vi "Chamber controller Dec 2 2016 new turbo - biased QCM.vi"() -> ()   [LabVIEW 2014]
uses:
  <vilib>/Instr/_visa.llb/VISA Configure Serial Port (Instr).vi
  Environmental Chamber LabVIEW and Instruments/Drivers and Software/Keithley 2100 Series/Public/Configure/Configure 2 Wire Resistance.vi
  <vilib>/Utility/file.llb/Write To Spreadsheet File (string).vi
  <vilib>/Utility/file.llb/Read From Spreadsheet File (string).vi
  Environmental Chamber LabVIEW and Instruments/Drivers and Software/keithley_6430/Keithley 6430/Public/Data/Read (Single Point).vi
  Environmental Chamber LabVIEW and Instruments/Drivers and Software/LabVIEW 8.2 Drivers/keithley_24xx/Keithley 24XX/Public/Data/Read (Single Point).vi
  Environmental Chamber LabVIEW and Instruments/Drivers and Software/keithley_24xx/Keithley 24XX/Keithley 24XX.lvlib
  Environmental Chamber LabVIEW and Instruments/Drivers and Software/keithley_6430/Keithley 6430/Keithley 6430.lvlib
  Environmental Chamber LabVIEW and Instruments/Drivers and Software/Keithley 2100 Series/Keithley 2100 Series.lvlib
panel:
  out "SRS freq plot":dbl(graph)
  out "Numeric bias":dbl
  out "bias voltage":string
  out "Current":sgl
  out "Resistance":sgl
  in  "Applied Voltage (V)":dbl min=-5.0 max=5.0 step=5e-06
  in  "Arduino COMs":T1={"Arduino 1"="COM23", "Arduino 2"="COM24", "Arduino 3"="COM25", "Arduino 4"="COM26", "Arduino 5"="COM27", "Arduino 6"="COM28"}
  out "saving data?":bool
  out "ArduinoQCM\ncluster":T2 caption="Arduino QCM" {"6" format="%_8g"; "5" format="%_8g"; "4" format="%_8g"; "3" format="%_8g"; "2" format="%_8g"; "1" format="%#_10g"}
  in  "Data logging settings":T3={"Save during sequence only"=TRUE, "Save now"=FALSE, "sec between data points"=0.0, "Current data file path"=path "", "Save sample names"={"QCM1"="", "QCM2"="", "QCM3"="", "QCM4"="", "QCM5"="", "QCM6"="", "SRS"="", "K-2420"="", "K-6430"="", "K-2100"=""}, "Experiment Notes"=""} {"sec between data points" min=0.0 max=30.0 format="%#_13g"}
  in  "Sequence cluster":T4={"Save sequence"=FALSE, "Clear sequence"=FALSE, "Import sequence file"=FALSE, "Tare elapsed time"=TRUE, "Run Sequence"=FALSE, "Stop program when sequence ends"=TRUE, "User-defined\nsequence"=[], "Sequence end time"="", "Sequence\npreview"=[], "Current\nstep"=0} caption="Sequence settings"
  in  "Pressure parameters cluster":T5={"valve % open"=100.0, "Desired pressure"=0.0, "Vapor sccm"=0.0, "Gas sccm"=0.0, "Valve mode"=enum."% Open", "Pressure Mode"=enum."Abs. pressure", "analyte partial pressure"=23.8, "Turbo pump\nauto on"=TRUE, "Valve position (%)"=0.0, "read pressure"=0.0, "read vapor flow"=0.0, "read gas flow"=0.0, "pressure chart"={"pressure"=0.0}} caption="Pressure settings" {"read gas flow" format="%#_3g"; "read vapor flow" format="%#_3g"; "read pressure" format="%#_7f"; "Valve position (%)" format="%#_3g"; "analyte partial pressure" min=0.0 max=100.0 step=5.0; "Gas sccm" min=0 max=200 step=5; "Vapor sccm" min=0 max=200 step=5; "Desired pressure" min=0.0 max=760.0 step=5.0; "valve % open" min=0.0 max=100.0 step=5.0 format="%#_2f"}
  out "J-KEM temp chart":dbl(graph)
  out "Elapsed time (min)":dbl
  out "State date/time":string caption="Start time"
  out "K-2100 (Ohm)":cluster{"Measurement":dbl}(graph) caption="K-2100"
  out "K-6430":cluster{"Measurement":dbl}(graph)
  out "K-2420":cluster{"Applied Voltage (V)":dbl}(graph)
  in  "Gate time (sec)":enum16{"0.1", "1.0 ", "10"}(ring)=enum."1.0 "
  out "Hz":dbl format="%#.7f"
  out "QCM plot":T6(graph)
  in  "Stop":bool
  in  "Clear all charts":bool
  out "O2 sensor output":dbl[](array[numeric]) caption="atm\nTorr"
  in  "rapidox O2 Sensor":bool
  in  "setnag O2 Pump":bool
  in  "Baud Rate 2":i32(ring)=2 items=["2400", "4800", "9600", "19200", "38400", "57600", "115200"]
  in  "Com Port":i32(ring) items=["Com 1", "Com 2", "Com 3", "Com 4", "Com 5", "Com 6", "COM 7", "COM 8", "COM 9", "COM 10", "COM 11", "COM 12", "com 13", "COM 14"]
  in  "Com Port 2":i32(ring) items=["Com 1", "Com 2", "Com 3", "Com 4", "Com 5", "Com 6", "COM 7", "COM 8", "COM 9", "COM 10", "COM 11", "COM 12", "com 13", "COM 14"]
  out "Waveform Chart":cluster{dbl}(graph)
  out "O2 Concentration (PPM)":dbl
  out "Waveform Chart 6":cluster{dbl}(graph)
  # "SRS"
  # "Currently Unused"
  # "100%"
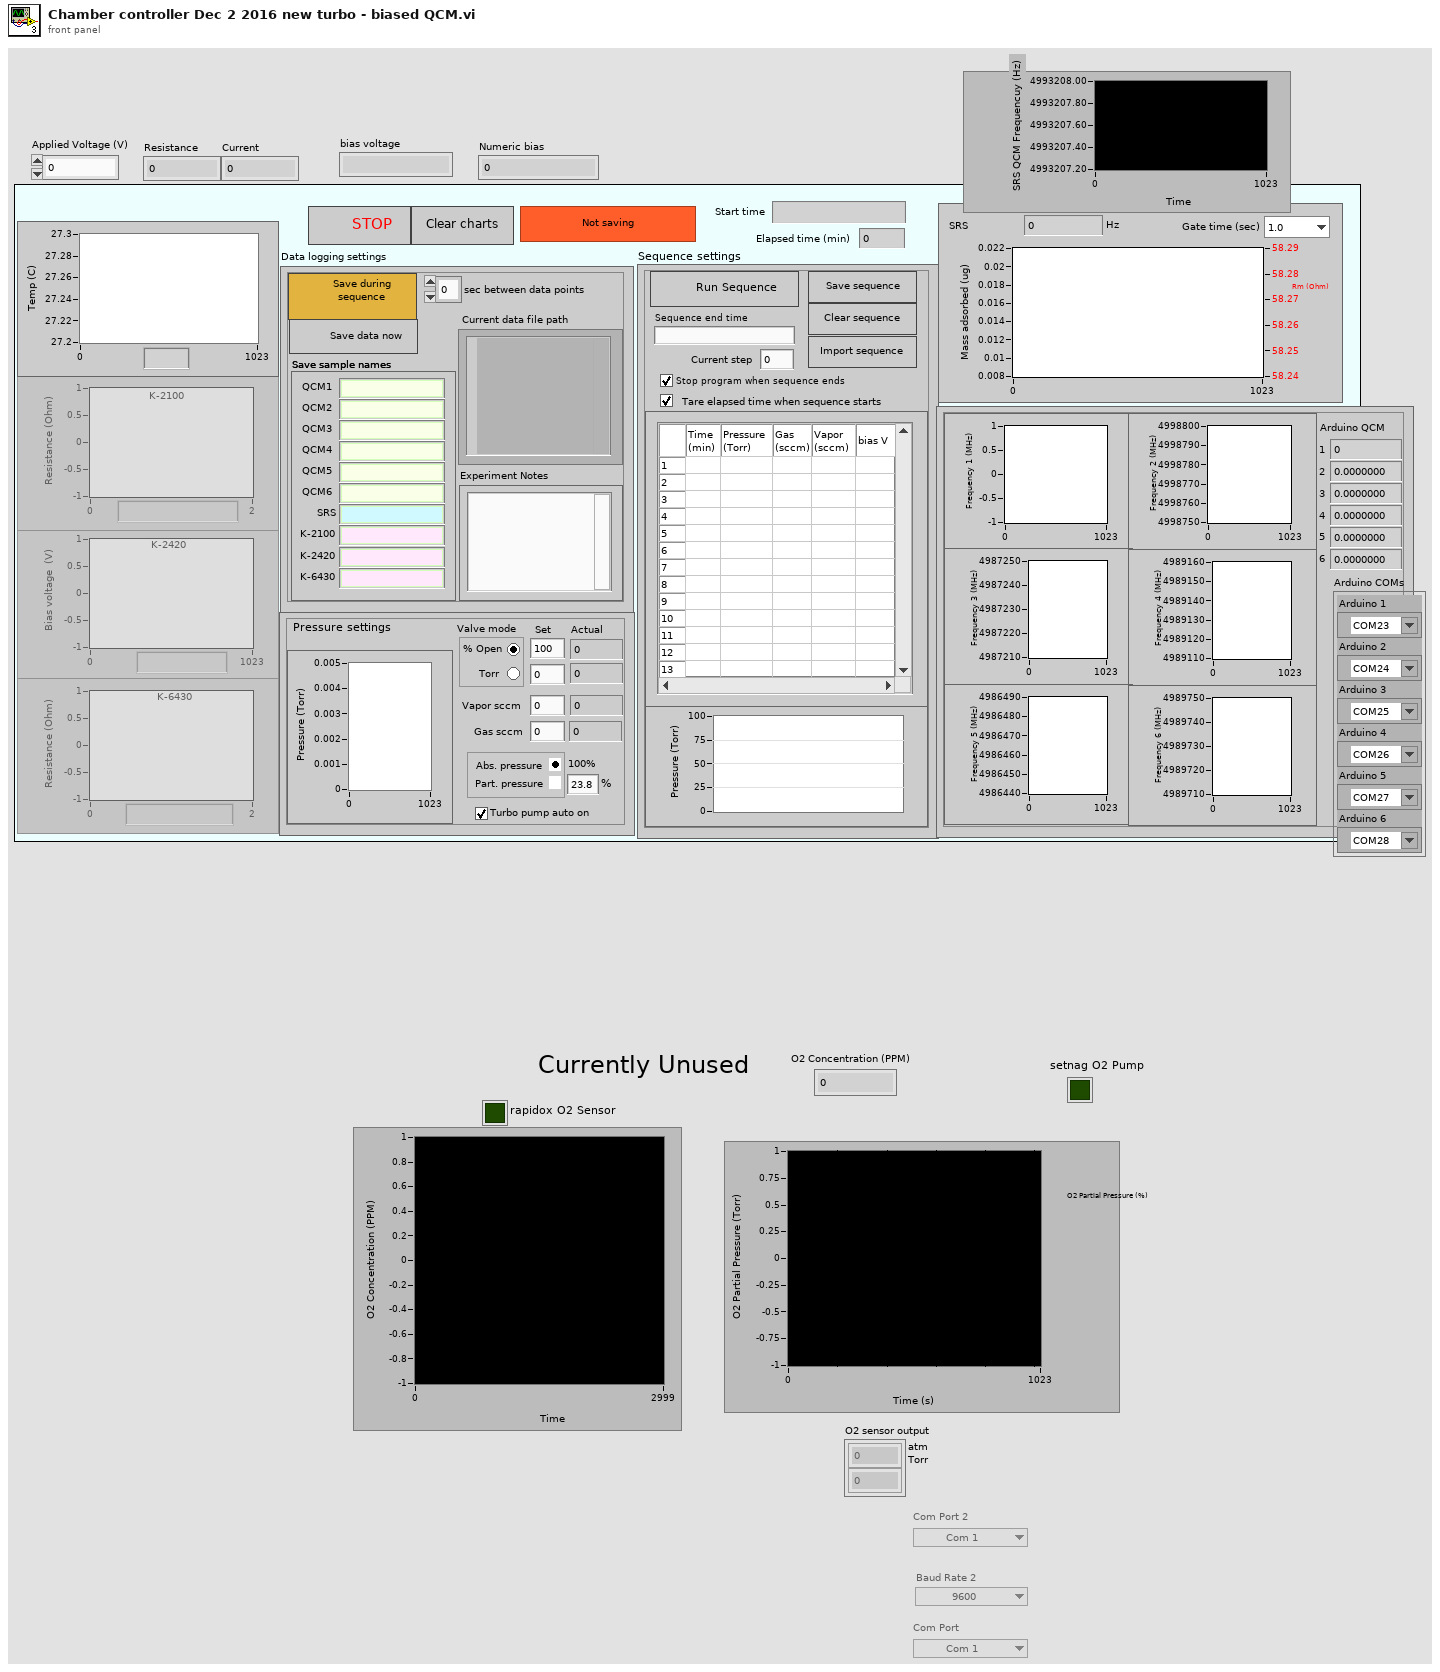
[diagram p1: front panel]
types:
  T1 = cluster{"Arduino 1":refnum<visa-resource-name>, "Arduino 2":refnum<visa-resource-name>, "Arduino 3":refnum<visa-resource-name>, "Arduino 4":refnum<visa-resource-name>, "Arduino 5":refnum<visa-resource-name>, "Arduino 6":refnum<visa-resource-name>}
  T2 = cluster{"arduino qcm 1":dbl, "1":dbl, "arduino qcm 2":dbl, "2":dbl, "arduino qcm 3":dbl, "3":dbl, "arduino qcm 4":dbl, "4":dbl, "arduino qcm 5":dbl, "5":dbl, "arduino qcm 6":dbl, "6":dbl}
  T3 = cluster{"Save during sequence only":bool, "Save now":bool, "sec between data points":dbl, "Current data file path":path, "Save sample names":cluster{"QCM1":string, "QCM2":string, "QCM3":string, "QCM4":string, "QCM5":string, "QCM6":string, "SRS":string, "K-2420":string, "K-6430":string, "K-2100":string}, "Experiment Notes":string}
  T4 = cluster{"Save sequence":bool, "Clear sequence":bool, "Import sequence file":bool, "Tare elapsed time":bool, "Run Sequence":bool, "Stop program when sequence ends":bool, "User-defined\nsequence":string[][], "Sequence end time":string, "Sequence\npreview":cluster{dbl[], dbl[]}[], "Current\nstep":i32}
  T5 = cluster{"valve % open":dbl, "Desired pressure":dbl, "Vapor sccm":sgl, "Gas sccm":sgl, "Valve mode":enum32{"% Open", "Torr "}, "Pressure Mode":enum32{"Abs. pressure", " Part. pressure"}, "analyte partial pressure":dbl, "Turbo pump\nauto on":bool, "Valve position (%)":dbl, "read pressure":dbl, "read vapor flow":dbl, "read gas flow":dbl, "pressure chart":cluster{"pressure":dbl}}
  T6 = cluster{"Numeric Control":dbl, "Resistance out":dbl}
  T7 = cluster{"Keithley 6430":bool, "J-KEM":bool, "Keithley 2420":bool, "Keithley 2100":bool, "SRS QCM":bool, "Pressure control":bool, "Arduino":bool}
  T8 = enum8{"Enabled", "Disabled", "Disabled and Grayed Out"}
  T9 = enum16{"open", "open or create", "create or replace", "create", "open (read only)"}
  T10 = enum16{"no parity", "odd parity", "even parity", "mark parity", "space parity"}
  T11 = cluster{"String":string, "String":string, "String":string}
  T12 = cluster{bool, "task out":refnum<k21>, "error out":errorcluster, "task out":refnum<k21>, "error out":errorcluster, "turbo pump":refnum<visa-resource-name>, "error out":errorcluster}
  T13 = cluster{bool, "task out":refnum<k21>, "error out":errorcluster, "task out":refnum<k21>, "error out":errorcluster, "VISA resource name out":refnum<visa-resource-name>, "error out":errorcluster}
  T14 = cluster{bool, "VISA resource name":refnum<visa-resource-name>, "error out":errorcluster}
  T15 = cluster{bool, "VISA resource name out":refnum<visa-resource-name>, "error out":errorcluster}
  T16 = cluster{"VISA resource name out":refnum<visa-resource-name>, "error out":errorcluster, "VISA resource name out":refnum<visa-resource-name>, "error out":errorcluster, "VISA resource name out":refnum<visa-resource-name>, "error out":errorcluster, "VISA resource name out":refnum<visa-resource-name>, "error out":errorcluster, "VISA resource name out":refnum<visa-resource-name>, "error out":errorcluster, "VISA resource name out 2":refnum<visa-resource-name>, "error out 2":errorcluster}
  T17 = cluster{"Boolean":bool, "VISA resource name out":refnum<visa-resource-name>, "error out":errorcluster}
  T18 = cluster{bool, "VISA out":refnum<visa-resource-name>, "error out":errorcluster}
  T19 = cluster{"Boolean":bool, "VISA out":refnum<visa-resource-name>, "error out":errorcluster}
  T20 = cluster{"Numeric Control":dbl, "Cluster":cluster{"Numeric Control":dbl}, "String":string, "error out":errorcluster}
  T21 = cluster{bool, "Com Port":i32, "Numeric Control out":dbl}
  T22 = cluster{"Arduino address":refnum<visa-resource-name>, "error in (no error)":errorcluster, "Arduino address 2":refnum<visa-resource-name>, "error in (no error) 2":errorcluster, "Arduino address 3":refnum<visa-resource-name>, "error in (no error) 3":errorcluster, "Arduino address 4":refnum<visa-resource-name>, "error in (no error) 4":errorcluster, "Arduino address 5":refnum<visa-resource-name>, "error in (no error) 5":errorcluster, "Arduino address 6":refnum<visa-resource-name>, "error in (no error) 6":errorcluster}
  T23 = cluster{"mean":string, "mean":string, "mean":string, "mean":string, "mean":string, "mean":string}
  T24 = cluster{"valve % open":dbl, "Desired pressure":dbl, "Vapor sccm":sgl, "Gas sccm":sgl, "Valve mode":enum32{"% Open", "Torr "}, "Pressure Mode":enum32{"Abs. pressure", " Part. pressure"}, "analyte partial pressure":dbl}
  T25 = cluster{"User-defined\nsequence":string[][], "Present (s)":dbl, "current  step # in":i32, "sequence end time in":timestamp}
  T26 = cluster{"current  step # in":i32, "sequence end time in":timestamp, "Boolean":bool}
  T27 = cluster{"press/RH/gas/vapor":cluster{"pressure":string, "RH":string, "gas flow":string, "vapor flow":string}, "Cluster":cluster{"Valve position (%)":dbl, "read pressure":dbl, "read vapor flow":dbl, "read gas flow":dbl}}
  T28 = cluster{"Boolean":bool, "task out":refnum<k21>, "error out":errorcluster, "task out":refnum<k21>, "error out":errorcluster, "VISA resource name out":refnum<visa-resource-name>, "error out":errorcluster}
  T29 = cluster{"f":dbl, "f":dbl, "f":dbl, "f":dbl, "f":dbl}[]
  T30 = cluster{"pressure":string, "RH":string, "gas flow":string, "vapor flow":string}
  T31 = cluster{"Valve position (%)":dbl, "read pressure":dbl, "read vapor flow":dbl, "read gas flow":dbl}
  T32 = cluster{"mean":dbl, "mean":dbl, "mean":dbl, "mean":dbl, "mean":dbl, "mean":dbl}
  T33 = cluster{"QCM1":string, "QCM2":string, "QCM3":string, "QCM4":string, "QCM5":string, "QCM6":string, "SRS":string, "K-2420":string, "K-6430":string, "K-2100":string}
  T34 = cluster{"mean":dbl, "mean":dbl, "mean":dbl, "mean":dbl, "mean":dbl, "mean":dbl, "mean":dbl, "mean":dbl, "mean":dbl, "mean":dbl, "mean":dbl, "mean":dbl}
  T35 = cluster{"String data out":string, string, string, string}
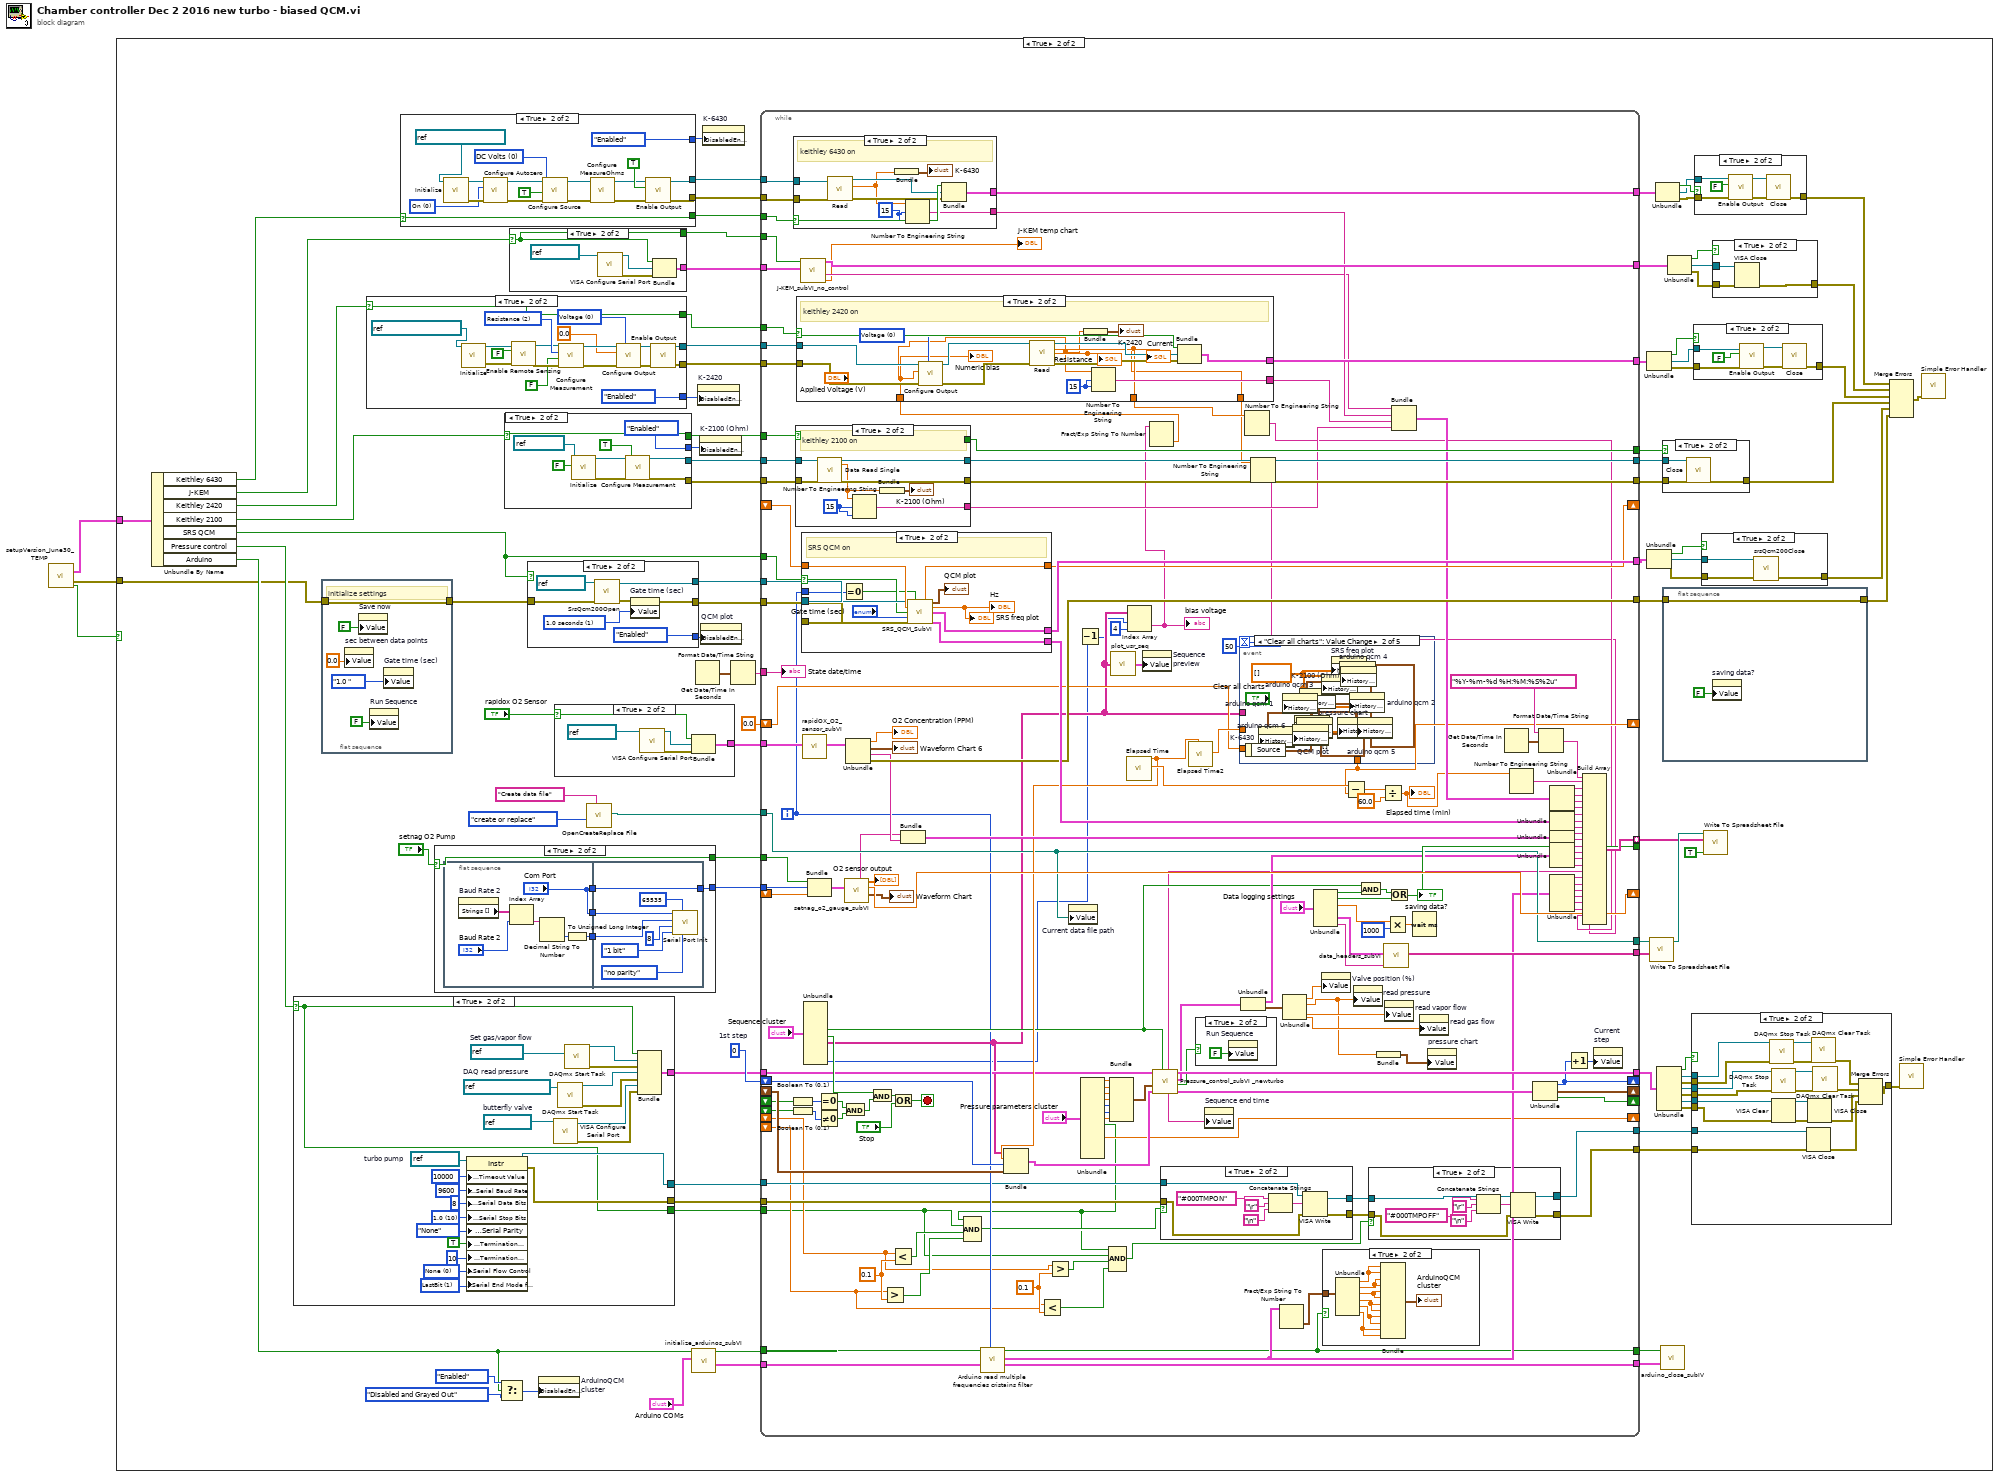
[diagram p0: block diagram]
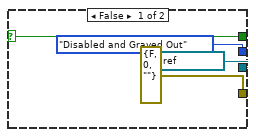
[diagram p4: hidden frame]
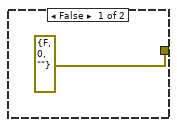
[diagram p5: hidden frame]
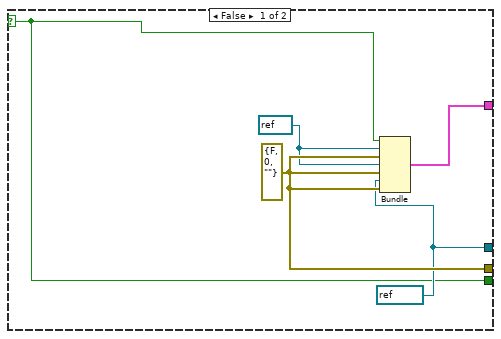
[diagram p6: hidden frame]
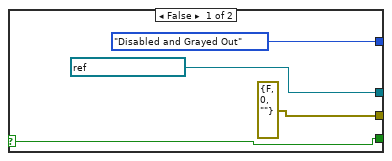
[diagram p8: hidden frame]
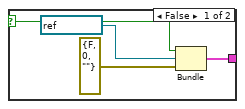
[diagram p9: hidden frame]
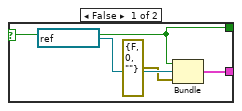
[diagram p11: hidden frame]
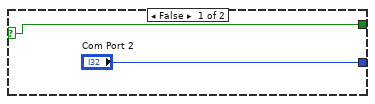
[diagram p12: hidden frame]
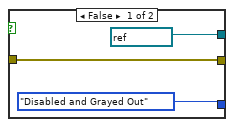
[diagram p14: hidden frame]
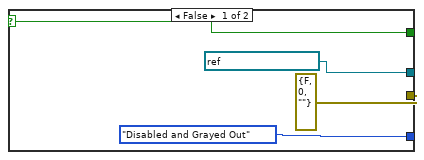
[diagram p16: hidden frame]
diagram:
  n1 = call "setupVersion_June30_TEMP.vi"() -> ("Instruments on/off"=w1:T7, "error IO"=w2:errorcluster, "OK"=w3:bool)  [unwired: 13 in]
  n2 = case shown="True" w3 {
    tunnel: w2 -> [_ w17]
    tunnel: w1 -> [_ w27]
    frame False {
    }
    frame True {
      w34 = 0  # 1st step
      n3 = Unbundle By Name(w27) -> ("Keithley 6430"=w26:bool, "J-KEM"=w25:bool, "Keithley 2420"=w24:bool, "Keithley 2100"=w23:bool, "SRS QCM"=w22:bool, "Pressure control"=w21:bool, "Arduino"=w20:bool)
      n4 = case shown="True" w21 {
        selector: w21 -> [w142 w147]
        tunnel: [w146 w148] -> w15
        tunnel: [w145 w150] -> w7
        tunnel: [w143 w149] -> w8
        tunnel: [w142 w147] -> w6
        frame False {
          w143 = refnum<visa-resource-name> refnum ("turbo pump")
          w144 = refnum<k21> refnum ("task out")
          w145 = errorcluster {"status"=FALSE, "code"=0, "source"=""} ("error out")
          n5 = Bundle(w142, "task out"=w144, "error out"=w145, "task out"=w144, "error out"=w145, "turbo pump"=w143, "error out"=w145) -> (w146:T12)  [unwired: 1 in]
        }
        frame True {
          w154 = u16 1 items=["None", "LastBit", "TermChar"] ("Serial Settings:Serial End Mode for Reads")
          w152 = u16 0 items=["None", "XON/XOFF", "RTS/CTS", "XON/XOFF & RTS/CTS", "DTR/DSR", "XON/XOFF & DTR/DSR"] ("flow control (0:none)")
          w155 = u16 10 items=["1.0"=10, "1.5"=15, "2.0"=20] ("stop bits (10: 1 bit)")
          w151 = refnum<visa-resource-name> "COM7"  # turbo pump
          w167 = refnum<visa-resource-name> "COM5"  # butterfly valve
          w168 = refnum<k21> "Setflow"  # Set gas/vapor flow
          w169 = refnum<k21> "AllDaqReadings"  # DAQ read pressure
          n6 = property class="Instr"(reference=w151, "General Settings:Timeout Value"=u32 10000 ("timeout (10sec)"), "Serial Settings:Serial Baud Rate"=u32 9600 ("baud rate (9600)"), "Serial Settings:Serial Data Bits"=u16 8 ("data bits (8)"), "Serial Settings:Serial Stop Bits"=w155, "Serial Settings:Serial Parity"=enum16{"None", "Odd", "Even", "Mark", "Space"}."None" ("parity (0:none)"), "Message Based Settings:Termination Character Enable"=TRUE ("Enable Termination\nChar (T)"), "Message Based Settings:Termination Character"=u8 10 ("termination char\n(0xA = '\\n' = LF)"), "Serial Settings:Serial Flow Control"=w152, "Serial Settings:Serial End Mode for Reads"=w154) -> (reference out=w149:refnum<visa-resource-name>, error out=w150:errorcluster)  [unwired: 1 in]
          n7 = call-poly "VISA Configure Serial Port"("VISA resource name"=w167) -> ("VISA resource name out"=w162:refnum<visa-resource-name>, "error out"=w161:errorcluster)  [unwired: 13 in]
          n8 = call <vilib>:"DAQmx Start Task.vi"("task/channels in"=w169) -> ("task out"=w164:refnum<k21>, "error out"=w163:errorcluster)  [unwired: 13 in]
          n9 = call <vilib>:"DAQmx Start Task.vi"("task/channels in"=w168) -> ("task out"=w166:refnum<k21>, "error out"=w165:errorcluster)  [unwired: 13 in]
          n10 = Bundle(w147, "task out"=w166, "error out"=w165, "task out"=w164, "error out"=w163, "VISA resource name out"=w162, "error out"=w161) -> (w148:T13)  [unwired: 1 in]
        }
      }
      n11 = flat-sequence {
        tunnel: [w98] -> w16
        tunnel: w17 -> [w98]
        frame #0 {
          # "initialize settings"
          n12 = property on="sec between data points" class="DigNum (strict)"("Value"=0.0) -> ()  [unwired: 2 in, 2 out]
          n13 = property on="Save now" class="Bool (strict)"("Value"=FALSE) -> ()  [unwired: 2 in, 2 out]
          n14 = property on="Run Sequence" class="Bool (strict)"("Value"=FALSE) -> ()  [unwired: 2 in, 2 out]
          n15 = property on="Gate time (sec)" class="Enum (strict)"("Value"=enum16{"0.1", "1.0 ", "10"}."1.0 " ("Gate time (sec)")) -> ()  [unwired: 2 in, 2 out]
        }
      }
      n16 = case shown="True" w24 {
        selector: w24 -> [w261 w265]
        tunnel: [refnum<visa-resource-name> "GPIB1::24::INSTR" ("VISA resource name") w274] -> w95
        tunnel: [errorcluster {"status"=FALSE, "code"=0, "source"=""} ("error out") w269] -> w94
        tunnel: [T8."Disabled and Grayed Out" ("Disabled") T8."Enabled" ("Disabled")] -> w58
        tunnel: [w261 w265] -> w51
        frame False {
        }
        frame True {
          w276 = u16 0 items=["Voltage", "Current"] ("Source Mode  (0: Voltage)")
          w281 = u16 2 items=["Volts", "Current", "Resistance"] ("Function (0: Volts)")
          n17 = call "Initialize.vi"("VISA resource name"=refnum<visa-resource-name> "GPIB1::24::INSTR") -> ("error out"=w270:errorcluster, "VISA resource name out"=w273:refnum<visa-resource-name>)  [unwired: 9 in]
          n18 = call "Enable Remote Sensing.vi"("error in (no error)"=w270, "Enable Remote Sensing (T: Enable)"=FALSE ("4-wire?"), "VISA resource name"=w273) -> ("error out"=w271:errorcluster, "VISA resource name out"=w272:refnum<visa-resource-name>)  [unwired: 7 in]
          n19 = call "Configure Measurement.vi"("error in (no error)"=w271, "Enable Auto Range (T:Enable)"=FALSE, "Function (0: Volts)"=w281, "VISA resource name"=w272) -> ("error out"=w280:errorcluster, "VISA resource name out"=w279:refnum<visa-resource-name>)  [unwired: 6 in]
          n20 = call "Configure Output.vi"("Source Mode  (0: Voltage)"=w276, "error in (no error)"=w280, "Output Level (0)"=0.0 ("Applied Voltage (V)"), "VISA resource name"=w279) -> ("error out"=w278:errorcluster, "VISA resource name out"=w277:refnum<visa-resource-name>)  [unwired: 6 in]
          n21 = call "Enable Output.vi"("error in (no error)"=w278, "VISA resource name"=w277) -> ("error out"=w269:errorcluster, "VISA resource name out"=w274:refnum<visa-resource-name>)  [unwired: 8 in]
        }
      }
      n22 = case shown="True" w26 {
        selector: w26 -> [w177 w181]
        tunnel: [refnum<visa-resource-name> "GPIB0::29::INSTR" ("VISA resource name") w192] -> w64
        tunnel: [errorcluster {"status"=FALSE, "code"=0, "source"=""} ("error out") w193] -> w63
        tunnel: [T8."Disabled and Grayed Out" ("Disabled") T8."Enabled" ("Disabled")] -> w57
        tunnel: [w177 w181] -> w50
        frame False {
        }
        frame True {
          w182 = u16 0 items=["DC Volts", "DC Current"] ("Source Function (0: DC Volts)")
          w189 = u16 0 items=["On", "Off", "Once"] ("Autozero  (0: On)")
          n23 = call "Initialize.vi"("VISA resource name"=refnum<visa-resource-name> "GPIB0::29::INSTR") -> ("error out"=w190:errorcluster, "VISA resource name out"=w191:refnum<visa-resource-name>)  [unwired: 4 in, 5 out]
          n24 = call "Configure Autozero.vi"("error in (no error)"=w190, "Autozero  (0: On)"=w189, "VISA resource name"=w191) -> ("error out"=w185:errorcluster, "VISA resource name out"=w187:refnum<visa-resource-name>)  [unwired: 7 in]
          n25 = call "Configure Source.vi"("error in (no error)"=w185, "Auto Range (T:Enable)"=TRUE, "Source Function (0: DC Volts)"=w182, "VISA resource name"=w187) -> ("error out"=w184:errorcluster, "VISA resource name out"=w186:refnum<visa-resource-name>)  [unwired: 6 in]
          n26 = call "Configure MeasureOhms.vi"("error in (no error)"=w184, "VISA resource name"=w186) -> ("error out"=w197:errorcluster, "VISA resource name out"=w195:refnum<visa-resource-name>)  [unwired: 4 in, 4 out]
          n27 = call "Enable Output.vi"("error in (no error)"=w197, "Enable Output (F:Off)"=TRUE ("Output (F:Off)"), "VISA resource name"=w195) -> ("error out"=w193:errorcluster, "VISA resource name out"=w192:refnum<visa-resource-name>)  [unwired: 7 out]
        }
      }
      n28 = case shown="True" "setnag O2 Pump" {
        selector: "setnag O2 Pump" -> [w220 w222]
        tunnel: ["Com Port 2" w223] -> w91
        tunnel: [w220 w222] -> w39
        frame False {
        }
        frame True {
          n29 = flat-sequence {
            tunnel: ["Com Port"] -> w226
            tunnel: [w228] -> w225
            tunnel: ["Com Port"] -> w224
            tunnel: w226 -> [w234]
            tunnel: w225 -> [w233]
            tunnel: w224 -> [w235]
            tunnel: [w235] -> w223
            frame #0 {
              n30 = property on="Baud Rate 2" class="Ring (strict)"() -> ("Strings []"=w230:string[])  [unwired: 2 in, 2 out]
              n31 = Index Array(array=w230, index="Baud Rate 2") -> (element=w231:string)
              n32 = Decimal String To Number(string=w231) -> (number=w229:i32)  [unwired: 2 in, 1 out]
              n33 = To Unsigned Long Integer(number=w229) -> (unsigned 32bit integer=w228:u32)
            }
            frame #1 {
              n34 = call <vilib>:"Serial Port Init.vi"("parity"=T10."no parity", "buffer size"=u16 65535, "stop bits"=enum16{"1 bit", "1.5 bits", "2 bits"}."1 bit", "data bits"=u16 8, "baud rate"=w233, "port number"=w234) -> ()  [unwired: 1 in, 1 out]
            }
          }
        }
      }
      n35 = Select(t=T8."Enabled" ("Disabled"), s=w20, f=T8."Disabled and Grayed Out" ("Disabled")) -> (s? t:f=w31:T8)
      n36 = case shown="True" w23 {
        selector: w23 -> [w110 w115]
        tunnel: [refnum<visa-resource-name> "K-2100" ("VISA resource name out") w118] -> w48
        tunnel: [errorcluster {"status"=FALSE, "code"=0, "source"=""} ("error out") w117] -> w47
        tunnel: [w110 w115] -> w46
        tunnel: [T8."Disabled and Grayed Out" ("Disabled") T8."Enabled" ("Disabled")] -> w41
        frame False {
        }
        frame True {
          n37 = call "Initialize.vi"("VISA resource name"=refnum<visa-resource-name> "K-2100", "Reset? (T: Reset)"=FALSE) -> ("VISA resource name out"=w119:refnum<visa-resource-name>, "error out"=w116:errorcluster)  [unwired: 16 in]
          n38 = call-poly "Configure Measurement.vi"("VISA resource name"=w119, "error in (no error)"=w116, "Auto Range? (T: Auto)"=TRUE) -> ("VISA resource name out"=w118:refnum<visa-resource-name>, "error out"=w117:errorcluster)  [unwired: 15 in]
        }
      }
      n39 = case shown="True" w25 {
        selector: w25 -> [w211 w216]
        tunnel: [w212 w217] -> w80
        tunnel: [w211 w216] -> w74
        frame False {
          n40 = Bundle(w211, "VISA resource name"=refnum<visa-resource-name> "COM3", "error out"=errorcluster {"status"=FALSE, "code"=0, "source"=""}) -> (w212:T14)  [unwired: 1 in]
        }
        frame True {
          n41 = call-poly "VISA Configure Serial Port"("VISA resource name"=refnum<visa-resource-name> "COM3") -> ("VISA resource name out"=w218:refnum<visa-resource-name>, "error out"=w215:errorcluster)  [unwired: 13 in]
          n42 = Bundle(w216, "VISA resource name out"=w218, "error out"=w215) -> (w217:T15)  [unwired: 1 in]
        }
      }
      n43 = case shown="True" w22 {
        tunnel: [refnum<visa-resource-name> "COM6" ("VISA in") w250] -> w93
        tunnel: [w245 w247] -> w92
        tunnel: w16 -> [w245 w252]
        tunnel: [T8."Disabled and Grayed Out" ("Disabled") T8."Enabled" ("Disabled")] -> w59
        frame False {
        }
        frame True {
          w249 = u16 1 items=["0.1 seconds", "1.0 seconds", "10.0 seconds"] ("Gate time")
          n44 = call "SrsQcm200Open.vi"("error in"=w252, "VISA in"=refnum<visa-resource-name> "COM6") -> ("error out"=w248:errorcluster, "VISA out"=w250:refnum<visa-resource-name>)  [unwired: 3 in]
          n45 = property on="Gate time (sec)" class="Enum (strict)"(error in=w248, "Value"=w249) -> (error out=w247:errorcluster)  [unwired: 1 in, 1 out]
        }
      }
      n46 = property on="ArduinoQCM\ncluster" class="Clust (strict)"("DisabledEnum"=w31) -> ()  [unwired: 2 in, 2 out]
      n47 = case shown="True" "rapidox O2 Sensor" {
        selector: "rapidox O2 Sensor" -> [w198 w203]
        tunnel: [w199 w204] -> w70
        frame False {
          n48 = Bundle(w198, "VISA resource name"=refnum<visa-resource-name> "COM7", "error out"=errorcluster {"status"=FALSE, "code"=0, "source"=""}) -> (w199:T14)  [unwired: 1 in]
        }
        frame True {
          n49 = call-poly "VISA Configure Serial Port"("VISA resource name"=refnum<visa-resource-name> "COM7") -> ("VISA resource name out"=w205:refnum<visa-resource-name>, "error out"=w202:errorcluster)  [unwired: 13 in]
          n50 = Bundle(w203, "VISA resource name out"=w205, "error out"=w202) -> (w204:T15)  [unwired: 1 in]
        }
      }
      n51 = call "OpenCreateReplace File.vi"("prompt"="Create data file", "function (open:0)"=T9."create or replace") -> ("new file path"=w49:path)  [unwired: 6 in, 3 out]
      n52 = call "initialize_arduinos_subVI.vi"("arduino 1-6 addresses"="Arduino COMs", "arduinos on?"=w20) -> ("arduino addresses/errors"=w35:T16, "arduinos on/off"=w55:bool)  [unwired: 8 in]
      n53 = Get Date/Time In Seconds() -> (seconds since 1Jan1904=w97:timestamp)
      n54 = property on="K-2420" class="WFChart (strict)"("DisabledEnum"=w58) -> ()  [unwired: 2 in, 2 out]
      n55 = property on="K-2100 (Ohm)" class="WFChart (strict)"("DisabledEnum"=w41) -> ()  [unwired: 2 in, 2 out]
      n56 = property on="QCM plot" class="WFChart (strict)"("DisabledEnum"=w59) -> ()  [unwired: 2 in, 2 out]
      n57 = property on="K-6430" class="WFChart (strict)"("DisabledEnum"=w57) -> ()  [unwired: 2 in, 2 out]
      n58 = Format Date/Time String(seconds (now)=w97) -> (date/time string=w38:string)  [unwired: 2 in]
      n59 = while {
        shift-right: [w452] -> _
        shift-left: _ -> [w383]
        tunnel: [w436] -> w56 mode=indexing if=w405
        tunnel: w51 -> [w441]
        tunnel: w95 -> [w451]
        tunnel: w94 -> [w450]
        tunnel: w93 -> [w449]
        tunnel: w92 -> [w448]
        tunnel: w22 -> [w447]
        tunnel: w39 -> [w385]
        tunnel: w91 -> [w386]
        tunnel: [w446] -> w88
        tunnel: [w445] -> w84
        tunnel: w80 -> [w444]
        tunnel: [w443] -> w79
        tunnel: w74 -> [w442]
        tunnel: w70 -> [w394]
        tunnel: [w390] -> w19
        tunnel: [w328] -> w69
        tunnel: w49 -> [w328]
        shift-right: [w434] -> _
        shift-left: _ -> [w435]
        tunnel: w64 -> [w440]
        tunnel: w63 -> [w439]
        tunnel: [w438] -> w62
        tunnel: [w405] -> _
        tunnel: w55 -> [w316]
        tunnel: w35 -> [w319]
        tunnel: [w315] -> w53
        tunnel: [w317] -> w54
        tunnel: [w422] -> w52
        tunnel: w50 -> [w417]
        tunnel: w48 -> [w404]
        tunnel: w47 -> [w403]
        tunnel: w46 -> [w402]
        tunnel: [w401] -> w45
        tunnel: [w400] -> w44
        tunnel: [w399] -> w43
        shift-right: [w377] -> _
        shift-left: 0.0 ("Elapsed Time (s)") -> [w378]
        tunnel: w38 -> [w368]
        tunnel: w15 -> [w312]
        shift-right: [w324] -> _
        shift-left: w34 -> [w341]
        shift-right: [w347] -> _
        shift-left: _ -> [w345]
        shift-right: [w346] -> _
        shift-left: _ -> [w344]
        shift-left: _ -> [w343]
        tunnel: [w339] -> w33
        tunnel: w8 -> [w307]
        tunnel: w7 -> [w306]
        tunnel: w6 -> [w296]
        tunnel: [w301] -> w5
        tunnel: [w302] -> w4
        shift-right: [w311] -> _
        shift-left: _ -> [w298]
        shift-left: _ -> [w297]
        i -> [w314]
        stop <- w407 stop-if-true
        w300 = 0.1 ("y")
        w310 = 0.1 ("y")
        n60 = Boolean To (0,1)(Boolean=w344) -> (0, 1=w415:i16)
        n61 = Boolean To (0,1)(Boolean=w343) -> (0, 1=w414:i16)
        n62 = case "Keithley 6430" shown="True" w417 {
          selector: w417 -> [w507 w518]
          tunnel: w440 -> [w506 w515]
          tunnel: w439 -> [w505 w514]
          tunnel: ["" w517] -> w389
          tunnel: [w504 w516] -> w438
          frame False {
            # "keithley 6430 off"
            n63 = Bundle(w507, "VISA resource name out"=w506, "error out"=w505) -> (w504:T15)  [unwired: 1 in]
          }
          frame True {
            w509 = i16 15 ("width (-)")
            # "keithley 6430 on"
            n64 = call-poly "Read.vi"("error in (no error)"=w514, "VISA resource name"=w515) -> ("error out"=w513:errorcluster, "Measurement"=w511:dbl, "VISA resource name out"=w512:refnum<visa-resource-name>)  [unwired: 1 in, 6 out]
            n65 = Bundle("Measurement"=w511) -> (→"K-6430":cluster{"Measurement":dbl})  [unwired: 1 in]
            n66 = Number To Engineering String(2:w509, 3:w509, 4:w511) -> (0:w517:string)  [unwired: 1 in]
            n67 = Bundle(w518, "VISA resource name out"=w512, "error out"=w513) -> (w516:T15)  [unwired: 1 in]
          }
        }
        n68 = case shown="True" w402 {
          selector: w402 -> [w483 w488]
          tunnel: [w484 w495] -> w400
          tunnel: [w485 w494] -> w399
          tunnel: w404 -> [w484 w493]
          tunnel: w403 -> [w485 w492]
          tunnel: ["" w490] -> w387
          tunnel: [w483 w488] -> w401
          frame False {
            # "keithley 2100 off"
          }
          frame True {
            w487 = i16 15 ("width (-)")
            # "keithley 2100 on"
            n69 = call "Data Read Single.vi"("VISA resource name"=w493, "error in (no error)"=w492) -> ("VISA resource name out"=w495:refnum<visa-resource-name>, "Measurement"=w491:dbl, "error out"=w494:errorcluster)  [unwired: 15 in]
            n70 = Number To Engineering String ("elapsed time (min)")(2:w487, 3:w487, 4:w491) -> (0:w490:string)  [unwired: 1 in]
            n71 = Bundle("Measurement"=w491) -> (→"K-2100 (Ohm)":cluster{"Measurement":dbl})  [unwired: 1 in]
          }
        }
        n72 = call "J-KEM_subVI_no_control.vi"("Address in"=w444, "J-KEM on?"=w442) -> ("Temp (C)"=→"J-KEM temp chart":dbl, "String data out"=w376:string, "Address out"=w443:T17)  [unwired: 6 in, 1 out]
        n73 = case "SRS QCM" shown="True" w447 {
          selector: w447 -> [w542 w551]
          tunnel: w449 -> [w545 w553]
          tunnel: w448 -> [w544 w554]
          tunnel: [w543 w557] -> w445
          tunnel: w435 -> [w540 w556]
          tunnel: [w540 w555] -> w434
          tunnel: [T11 {"String"="", "String"="", "String"=""} ("M,F,MR output cluster") w550] -> w427
          tunnel: w314 -> [_ w547]
          frame False {
            # "SRS QCM off"
            n74 = Bundle(w542, "VISA out"=w545, "error out"=w544) -> (w543:T18)  [unwired: 1 in]
          }
          frame True {
            # "SRS QCM on"
            n75 = Equal To 0?(x=w547) -> (x = 0?=w548:bool)
            n76 = call "SRS_QCM_SubVI.vi"("VISA Refnum in"=w553, "first iteration?"=w548, "Frequency out 3"=w556, "Boolean 2"=w551, "Gate time"="Gate time (sec)", "error in (no error)"=w554) -> ("Frequency out 2"=w555:dbl, "Cluster"=→"QCM plot":T6, "Frequency out"=→"Hz" →"SRS freq plot":dbl, "Cluster 2"=w557:T19, "M,F,MR output cluster"=w550:T11)  [unwired: 2 in, 3 out]
          }
        }
        n77 = call "rapidOX_O2_sensor_subVI.vi"("rapid ox info in"=w394) -> ("rapidox info out"=w393:T20)  [unwired: 10 in]
        n78 = Unbundle("Sequence cluster") -> ("Run Sequence"=w334:bool, "Stop program when sequence ends"=w342:bool, "User-defined\nsequence"=w292:string[][], "Current\nstep"=w290:i32)  [unwired: 6 out]
        n79 = Bundle(w385, "Com Port"=w386, "Numeric Control out"=w383) -> (w384:T21)  [unwired: 1 in]
        n80 = Equal To 0?(x=w415) -> (x = 0?=w412:bool)
        n81 = Not Equal To 0?(x=w414) -> (x != 0?=w413:bool)
        n82 = And(x=w412, y=w413) -> (x .and. y?=w406:bool)
        n83 = call "setnag_o2_gauge_subVI.vi"("setnag info in"=w384) -> ("Cluster"=→"Waveform Chart":cluster{"Numeric Control":dbl}, "Numeric Control out"=w452:dbl, "Array"=→"O2 sensor output":dbl[], "String"=w325:string)  [unwired: 7 in]
        n84 = Unbundle(w393) -> ("Numeric Control"=→"O2 Concentration (PPM)":dbl, "Cluster"=→"Waveform Chart 6":cluster{"Numeric Control":dbl}, "String"=w367:string, "error out"=w390:errorcluster)
        n85 = And(x=w342, y=w406) -> (x .and. y?=w381:bool)
        n86 = Greater?(x=w297, y=w310) -> (0:w309:bool)
        n87 = Less?(x=w298, y=w310) -> (x < y?=w308:bool)
        n88 = Or(x=w381, y="Stop") -> (x .or. y?=w407:bool)
        n89 = Bundle("String"=w325, "String"=w367) -> (w366:cluster{"String":string, "String":string})  [unwired: 1 in]
        n90 = call "Arduino read multiple frequencies cristains filter.vi"("main loop iteration number"=w314, "arduino addresses in"=w319, "arduinos on?"=w316) -> ("arduino addresses out"=w317:T22, "arduino frequencies out"=w318:T23, "arduinos on"=w315:bool)  [unwired: 6 in]
        n91 = Less?(x=w297, y=w300) -> (x < y?=w294:bool)
        n92 = Greater?(x=w298, y=w300) -> (0:w295:bool)
        n93 = property on="Current data file path" class="Path"("Value"=w328) -> ()  [unwired: 2 in, 2 out]
        n94 = Decrement(x=w290) -> (x-1=w289:i32)
        n95 = Unbundle("Pressure parameters cluster") -> ("valve % open"=w356:dbl, "Desired pressure"=w358:dbl, "Vapor sccm"=w359:sgl, "Gas sccm"=w360:sgl, "Valve mode"=w361:enum32{"% Open", "Torr "}, "Pressure Mode"=w362:enum32{"Abs. pressure", " Part. pressure"}, "analyte partial pressure"=w363:dbl, "Turbo pump\nauto on"=w299:bool, "read pressure"=w311:dbl)  [unwired: 4 out]
        n96 = Compound Arithmetic op=AND(w299, w296, w308, w309) -> (w305:bool)
        n97 = Compound Arithmetic op=AND(w299, w296, w295, w294) -> (w293:bool)
        n98 = Bundle("valve % open"=w356, "Desired pressure"=w358, "Vapor sccm"=w359, "Gas sccm"=w360, "Valve mode"=w361, "Pressure Mode"=w362, "analyte partial pressure"=w363) -> (w355:T24)  [unwired: 1 in]
        n99 = call "plot_usr_seq.vi"("User-defined sequence"=w292) -> ("Sequence Preview"=w330:cluster{dbl[], dbl[]}[])
        n100 = call "Elapsed Time"() -> ("Present (s)"=w349:dbl, "Elapsed Time (s)"=w396:dbl)  [unwired: 12 in, 6 out]
        n101 = Bundle("User-defined\nsequence"=w292, "Present (s)"=w349, "current  step # in"=w341, "sequence end time in"=w345) -> (w350:T25)  [unwired: 1 in]
        n102 = Index Array(array=w292, index (row)=w289, index (col)=4 ("disabled index (col)")) -> (element=w288:string)
        "bias voltage" <- w288
        n103 = property on="Sequence\npreview" class="XYGraph (strict)"("Value"=w330) -> ()  [unwired: 2 in, 2 out]
        n104 = Fract/Exp String To Number(string=w288) -> (number=w283:dbl)  [unwired: 3 in, 1 out]
        n105 = case "Keithley 2420" shown="True" w441 {
          selector: w441 -> [w523 w537]
          tunnel: w451 -> [w522 w531]
          tunnel: w450 -> [w521 w528]
          tunnel: [w520 w535] -> w446
          tunnel: ["" w534] -> w388
          tunnel: w283 -> [_ w525]
          tunnel: [w519 w527] -> w287
          tunnel: [w519 w526] -> w286
          frame False {
            w519 = sgl 0.0 ("Current")
            # "keithley 2420 off"
            n106 = Bundle(w523, "VISA resource name out"=w522, "error out"=w521) -> (w520:T15)  [unwired: 1 in]
          }
          frame True {
            w532 = u16 0 items=["Voltage", "Current"] ("Source Mode  (0: Voltage)")
            w533 = i16 15 ("width (-)")
            # "keithley 2420 on"
            n107 = call "Configure Output.vi"("Source Mode  (0: Voltage)"=w532, "error in (no error)"=w528, "Output Level (0)"=w525, "VISA resource name"=w531) -> ("error out"=w529:errorcluster, "VISA resource name out"=w530:refnum<visa-resource-name>)  [unwired: 6 in]
            n108 = call-poly "Read.vi"("VISA resource name"=w530, "error in (no error)"=w529) -> ("VISA resource name out"=w538:refnum<visa-resource-name>, "Current"=w527:sgl, "Resistance"=w526:sgl, "error out"=w536:errorcluster)  [unwired: 7 in, 3 out]
            "Resistance" <- w526
            "Current" <- w527
            n109 = Bundle(w525) -> (→"K-2420":cluster{dbl})  [unwired: 1 in]
            n110 = Number To Engineering String(2:w533, 3:w533, 4:w525) -> (0:w534:string)  [unwired: 1 in]
            n111 = Bundle(w537, "VISA resource name out"=w538, "error out"=w536) -> (w535:T15)  [unwired: 1 in]
            "Numeric bias" <- w525
          }
        }
        n112 = call "Pressure_control_subVI _newturbo.vi"("Run Sequence"=w334, "user sequence, present (s) in, current step in, seq time in"=w350, "pressure parameters in"=w355, "pressure control on?/daq IDs/errors"=w312) -> ("current step # out, shift register time out, seq button on?"=w348:T26, "sequence over? USE THIS TO REINITIALIZE RUN SEQUENCE BUTTON SO PROGRAM ENDS"=w338:bool, "save press/RH/gasflow/vaporflow - read valve position/pressure/vaporflow/gasflow"=w337:T27, "pressure control on?/daq IDs/errors out"=w339:T28, "sequence end date/time string"=w340:string, "pressure_setpoint"=w321:string)  [unwired: 2 in]
        n113 = case shown="True" w305 {
          tunnel: w307 -> [w465 w468]
          tunnel: w306 -> [w464 w469]
          tunnel: [w465 w467] -> w304
          tunnel: [w464 w466] -> w303
          frame False {
          }
          frame True {
            n114 = Concatenate Strings("#000TMPON" ("write buffer 2"), "\r", "\n") -> (w470:string)
            n115 = VISA Write(VISA resource name=w468, write buffer=w470, error in (no error)=w469) -> (VISA resource name out=w467:refnum<visa-resource-name>, error out=w466:errorcluster)  [unwired: 1 out]
          }
        }
        n116 = call "Elapsed Time2"("Set Start Time (s)"=w349) -> ("Elapsed Time (s)"=w379:dbl)  [unwired: 11 in, 7 out]
        n117 = case shown="True" w338 {
          frame False {
          }
          frame True {
            n118 = property on="Run Sequence" class="Bool (strict)"("Value"=FALSE ("Run Sequence")) -> ()  [unwired: 2 in, 2 out]
          }
        }
        n119 = property on="Sequence end time" class="Str"("Value"=w340) -> ()  [unwired: 2 in, 2 out]
        n120 = event shown="[1] \"Clear all charts\": Value Change" {
          selector: _ -> [_ _ _ _ _]
          dyn-events: _ -> [_ _ _ _ _]
          timeout: 50 -> [_ _ _ _ _]
          tunnel: w292 -> [_ _ _ w502 _]
          tunnel: w379 -> [_ _ _ _ _]
          tunnel: w378 -> [w496 _ _ _ _]
          tunnel: [w496 _ _ _ _] -> w377
          event Timeout {
            n121 = event-data() -> ()  [unwired: 1 in, 1 out]
          }
          event "Clear all charts": Value Change {
            (unwired) T29 [] ("History Data")
            w499 = cluster{dbl}[] [] ("History Data")
            w500 = cluster{"Resistance":sgl}[] [] ("History Data")
            w497 = dbl[] [] ("History Data")
            n122 = event-data() -> ()  [unwired: 1 in, 1 out]
            n123 = property on="K-6430" class="WFChart (strict)"("History Data"=w500) -> ()  [unwired: 2 in, 2 out]
            n124 = property on="arduino qcm 1" class="WFChart (strict)"("History Data"=w497) -> ()  [unwired: 2 in, 2 out]
            n125 = property on="Waveform Chart" class="WFChart (strict)"("History Data"=w499) -> ()  [unwired: 2 in, 2 out]
            n126 = property on="arduino qcm 6" class="WFChart (strict)"("History Data"=w497) -> ()  [unwired: 2 in, 2 out]
            n127 = property on="QCM plot" class="WFChart (strict)"("History Data"=cluster{dbl, "Resistance out":dbl}[] []) -> ()  [unwired: 2 in, 2 out]
            n128 = property on="K-2100 (Ohm)" class="WFChart (strict)"("History Data"=w500) -> ()  [unwired: 2 in, 2 out]
            n129 = property on="arduino qcm 3" class="WFChart (strict)"("History Data"=w497) -> ()  [unwired: 2 in, 2 out]
            n130 = property on="SRS freq plot" class="WFChart (strict)"("History Data"=w497) -> ()  [unwired: 2 in, 2 out]
            n131 = property on="pressure chart" class="WFChart (strict)"("History Data"=w499) -> ()  [unwired: 2 in, 2 out]
            n132 = property on="arduino qcm 4" class="WFChart (strict)"("History Data"=w497) -> ()  [unwired: 2 in, 2 out]
            n133 = property on="K-2420" class="WFChart (strict)"("History Data"=w500) -> ()  [unwired: 2 in, 2 out]
            n134 = property on="arduino qcm 2" class="WFChart (strict)"("History Data"=w497) -> ()  [unwired: 2 in, 2 out]
            n135 = property on="arduino qcm 5" class="WFChart (strict)"("History Data"=w497) -> ()  [unwired: 2 in, 2 out]
          }
          event "Sequence cluster.Clear sequence": Value Change {
            n136 = event-data() -> ()  [unwired: 1 in, 1 out]
            n137 = property on="User-defined\nsequence" class="Tbl (strict)"("Value"=string[][] []) -> ()  [unwired: 2 in, 2 out]
          }
          event "Sequence cluster.Save sequence": Value Change {
            n138 = event-data() -> ()  [unwired: 1 in, 1 out]
            n139 = call-poly <vilib>:"Write To Spreadsheet File.vi"("2D data"=w502) -> ()  [unwired: 7 in, 1 out]
          }
          event "Sequence cluster.Import sequence file": Value Change {
            n140 = event-data() -> ()  [unwired: 1 in, 1 out]
            n141 = call-poly <vilib>:"Read From Spreadsheet File.vi"() -> ("all rows"=w503:string[][])  [unwired: 7 in, 4 out]
            n142 = property on="User-defined\nsequence" class="Tbl (strict)"("Value"=w503) -> ()  [unwired: 2 in, 2 out]
          }
        }
        n143 = Unbundle(w337) -> ("press/RH/gas/vapor"=w336:T30, "Cluster"=w335:T31)
        n144 = Number To Engineering String(4:w287) -> (0:w285:string)  [unwired: 3 in]
        n145 = Number To Engineering String(4:w286) -> (0:w284:string)  [unwired: 3 in]
        n146 = Fract/Exp String To Number(string=w318) -> (number=w313:T32)  [unwired: 3 in, 1 out]
        n147 = Unbundle(w335) -> ("Valve position (%)"=w333:dbl, "read pressure"=w327:dbl, "read vapor flow"=w332:dbl, "read gas flow"=w331:dbl)
        n148 = Unbundle("Data logging settings") -> ("Save during sequence only"=w409:bool, "Save now"=w411:bool, "sec between data points"=w398:dbl, "Save sample names"=w353:T33, "Experiment Notes"=w352:string)  [unwired: 1 out]
        n149 = property on="Valve position (%)" class="DigNum (strict)"("Value"=w333) -> ()  [unwired: 2 in, 2 out]
        n150 = case shown="True" w315 {
          tunnel: w313 -> [_ w482]
          frame False {
          }
          frame True {
            n151 = Unbundle(w482) -> ("mean"=w481:dbl, "mean"=w480:dbl, "mean"=w479:dbl, "mean"=w478:dbl, "mean"=w477:dbl, "mean"=w475:dbl)
            n152 = Bundle("mean"=w481, "mean"=w481, "mean"=w480, "mean"=w480, "mean"=w479, "mean"=w479, "mean"=w478, "mean"=w478, "mean"=w477, "mean"=w477, "mean"=w475, "mean"=w475) -> (→"ArduinoQCM\ncluster":T34)  [unwired: 1 in]
          }
        }
        n153 = Subtract(x=w396, y=w377) -> (x-y=w395:dbl)
        n154 = property on="read pressure" class="DigNum (strict)"("Value"=w327) -> ()  [unwired: 2 in, 2 out]
        n155 = And(x=w334, y=w409) -> (x .and. y?=w408:bool)
        n156 = case shown="True" w293 {
          tunnel: w304 -> [w455 w458]
          tunnel: w303 -> [w454 w459]
          tunnel: [w455 w457] -> w301
          tunnel: [w454 w456] -> w302
          frame False {
          }
          frame True {
            n157 = Concatenate Strings("#000TMPOFF" ("write buffer 2"), "\r", "\n") -> (w460:string)
            n158 = VISA Write(VISA resource name=w458, write buffer=w460, error in (no error)=w459) -> (VISA resource name out=w457:refnum<visa-resource-name>, error out=w456:errorcluster)  [unwired: 1 out]
          }
        }
        n159 = Bundle("read pressure"=w327) -> (w326:cluster{"read pressure":dbl})  [unwired: 1 in]
        n160 = Divide(x=w395, y=60.0) -> (x/y=w369:dbl)
        "Elapsed time (min)" <- w369
        n161 = call "data_headers_subVI.vi"("Experiment Notes"=w352, "Sample names"=w353) -> ("data headers"=w422:string[])  [unwired: 9 in]
        n162 = property on="read vapor flow" class="DigNum (strict)"("Value"=w332) -> ()  [unwired: 2 in, 2 out]
        n163 = Multiply(x=w398, y=u32 1000 ("x")) -> (x*y=w431:dbl)
        n164 = Or(x=w408, y=w411) -> (x .or. y?=w405:bool)
        "saving data?" <- w405
        n165 = Bundle("String data out"=w376, w389, w388, w387) -> (w382:T35)  [unwired: 1 in]
        n166 = Wait (ms)(milliseconds to wait=w431) -> ()  [unwired: 1 out]
        n167 = property on="read gas flow" class="DigNum (strict)"("Value"=w331) -> ()  [unwired: 2 in, 2 out]
        n168 = property on="pressure chart" class="WFChart (strict)"("Value"=w326) -> ()  [unwired: 2 in, 2 out]
        n169 = Get Date/Time In Seconds() -> (seconds since 1Jan1904=w453:timestamp)
        n170 = Number To Engineering String ("elapsed time (min)")(4:w369) -> (0:w374:string)  [unwired: 3 in]
        n171 = Unbundle(w348) -> ("current  step # in"=w324:i32, "sequence end time in"=w347:timestamp, "Boolean"=w346:bool)
        n172 = Format Date/Time String(time format string (%c)="%Y-%m-%d %H:%M:%S%2u", seconds (now)=w453) -> (date/time string=w428:string)  [unwired: 1 in]
        n173 = Unbundle(w382) -> ("String data out"=w373:string, w372:string, w371:string, w370:string)
        n174 = Unbundle(w427) -> ("String"=w375:string, "String"=w430:string, "String"=w429:string)
        n175 = Unbundle(w366) -> ("String"=w365:string, "String"=w364:string)
        n176 = Unbundle(w336) -> ("pressure"=w421:string, "RH"=w420:string, "gas flow"=w419:string, "vapor flow"=w418:string)
        n177 = Unbundle ("arduino 1-6")(w318) -> ("mean"=w322:string, "mean"=w426:string, "mean"=w425:string, "mean"=w424:string, "mean"=w423:string, "mean"=w320:string)
        n178 = Increment(x=w324) -> (x+1=w323:i32)
        n179 = Build Array(w428, w374, w373, w372, w371, w370, w375, w430, w429, w365, w364, w421, w420, w419, w418, w321, w322, w426, w425, w424, w423, w320, w285, w284) -> (w436:string[])
        n180 = property on="Current\nstep" class="DigNum (strict)"("Value"=w323) -> ()  [unwired: 2 in, 2 out]
        "State date/time" <- w368
      }
      n181 = Unbundle(w88) -> (w87:bool, "VISA resource name out"=w86:refnum<visa-resource-name>, "error out"=w85:errorcluster)
      n182 = Unbundle(w84) -> ("Boolean"=w83:bool, "VISA out"=w82:refnum<visa-resource-name>, "error out"=w81:errorcluster)
      n183 = call-poly <vilib>:"Write To Spreadsheet File.vi"("1D data"=w52, "file path (dialog if empty)"=w69) -> ("new file path (Not A Path if cancelled)"=w73:path)  [unwired: 6 in]
      n184 = Unbundle(w62) -> (w67:bool, "VISA resource name out"=w66:refnum<visa-resource-name>, "error out"=w65:errorcluster)
      n185 = Unbundle(w33) -> ("Boolean"=w32:bool, "task out"=w14:refnum<k21>, "error out"=w13:errorcluster, "task out"=w12:refnum<k21>, "error out"=w11:errorcluster, "VISA resource name out"=w10:refnum<visa-resource-name>, "error out"=w9:errorcluster)
      n186 = call "arduino_close_subIV.vi"("arduino 1-6 addresses and errors out"=w54, "arduinos on?"=w53) -> ()  [unwired: 10 in]
      n187 = case shown="True" w45 {
        tunnel: w44 -> [_ w108]
        tunnel: w43 -> [w105 w107]
        tunnel: [w105 w106] -> w42
        frame False {
        }
        frame True {
          n188 = call "Close.vi"("VISA resource name"=w108, "error in (no error)"=w107) -> ("error out"=w106:errorcluster)  [unwired: 17 in]
        }
      }
      n189 = flat-sequence {
        tunnel: w19 -> [w104]
        tunnel: [w104] -> w18
        frame #0 {
          n190 = property on="saving data?" class="Bool (strict)"("Value"=FALSE ("saving data?")) -> ()  [unwired: 2 in, 2 out]
        }
      }
      n191 = Unbundle(w79) -> ("Boolean"=w78:bool, "VISA resource name out"=w77:refnum<visa-resource-name>, "error out"=w76:errorcluster)
      n192 = case shown="True" w32 {
        tunnel: [errorcluster {"status"=FALSE, "code"=0, "source"=""} ("error out") w133] -> w37
        tunnel: w14 -> [_ w132]
        tunnel: w13 -> [_ w131]
        tunnel: w12 -> [_ w130]
        tunnel: w11 -> [_ w127]
        tunnel: w10 -> [_ w128]
        tunnel: w9 -> [_ w129]
        tunnel: w5 -> [_ w124]
        tunnel: w4 -> [_ w123]
        frame False {
        }
        frame True {
          n193 = call <vilib>:"DAQmx Stop Task.vi"("task/channels in"=w132, "error in"=w131) -> ("task out"=w139:refnum<k21>, "error out"=w138:errorcluster)  [unwired: 12 in]
          n194 = call <vilib>:"DAQmx Stop Task.vi"("task/channels in"=w130, "error in"=w127) -> ("task out"=w140:refnum<k21>, "error out"=w141:errorcluster)  [unwired: 12 in]
          n195 = VISA Clear(VISA resource name=w128, error in (no error)=w129) -> (VISA resource name out=w137:refnum<visa-resource-name>, error out=w136:errorcluster)
          n196 = VISA Close(VISA resource name=w124, error in (no error)=w123) -> (error out=w125:errorcluster)
          n197 = VISA Close(VISA resource name=w137, error in (no error)=w136) -> (error out=w126:errorcluster)
          n198 = call <vilib>:"DAQmx Clear Task.vi"("task in"=w139, "error in"=w138) -> ("error out"=w135:errorcluster)  [unwired: 13 in]
          n199 = call <vilib>:"DAQmx Clear Task.vi"("task in"=w140, "error in"=w141) -> ("error out"=w134:errorcluster)  [unwired: 13 in]
          n200 = Merge Errors(w135, w134, w126, w125) -> (w133:errorcluster)
        }
      }
      n201 = case shown="True" w87 {
        tunnel: w86 -> [_ w257]
        tunnel: w85 -> [w254 w256]
        tunnel: [w254 w255] -> w89
        frame False {
        }
        frame True {
          n202 = call "Enable Output.vi"("error in (no error)"=w256, "Enable Output (T: Enable)"=FALSE, "VISA resource name"=w257) -> ("error out"=w258:errorcluster, "VISA resource name out"=w260:refnum<visa-resource-name>)  [unwired: 7 in]
          n203 = call "Close.vi"("error in (no error)"=w258, "VISA resource name"=w260) -> ("error out"=w255:errorcluster)  [unwired: 9 in]
        }
      }
      n204 = case shown="True" w67 {
        tunnel: w66 -> [_ w172]
        tunnel: w65 -> [w170 w171]
        tunnel: [w170 w173] -> w61
        frame False {
        }
        frame True {
          n205 = call "Enable Output.vi"("error in (no error)"=w171, "Enable Output (F:Off)"=FALSE ("Output (F:Off)"), "VISA resource name"=w172) -> ("error out"=w174:errorcluster, "VISA resource name out"=w175:refnum<visa-resource-name>)  [unwired: 7 out]
          n206 = call "Close.vi"("error in (no error)"=w174, "VISA resource name"=w175) -> ("error out"=w173:errorcluster)  [unwired: 9 out]
        }
      }
      n207 = case shown="True" w83 {
        tunnel: w81 -> [w240 w243]
        tunnel: [w240 w242] -> w90
        tunnel: w82 -> [_ w241]
        frame False {
        }
        frame True {
          n208 = call "srsQcm200Close.vi"("error in"=w243, "Visa in"=w241) -> ("error out"=w242:errorcluster)  [unwired: 3 in]
        }
      }
      n209 = call-poly <vilib>:"Write To Spreadsheet File.vi"("append to file? (new file:F)"=TRUE, "2D data"=w56, "file path (dialog if empty)"=w73) -> ()  [unwired: 5 in, 1 out]
      n210 = case shown="True" w78 {
        tunnel: w77 -> [_ w210]
        tunnel: w76 -> [w207 w209]
        tunnel: [w207 w208] -> w75
        frame False {
        }
        frame True {
          n211 = VISA Close(VISA resource name=w210, error in (no error)=w209) -> (error out=w208:errorcluster)
        }
      }
      n212 = Merge Errors(w61, w75, w89, w42, w90, w18) -> (w96:errorcluster)
      n213 = call <vilib>:"Simple Error Handler.vi"("error in (no error)"=w37) -> ()  [unwired: 4 in, 5 out]
      n214 = call <vilib>:"Simple Error Handler.vi"("error in (no error)"=w96) -> ()  [unwired: 4 in, 5 out]
    }
  }
